vi "EnqueExperiment.vi"(0 "object in":refnum<class "Experiment.lvclass">, 1 "Message":string, 3 "Message Data":variant, 5 "error in (no error)":errorcluster) -> (14 "object out":refnum<class "Experiment.lvclass">, 19 "error out":errorcluster)   [LabVIEW 2023, in "Experiment.lvclass"]
uses:
  Experiment.lvclass
  Experiment.lvclass/Experiment.ctl
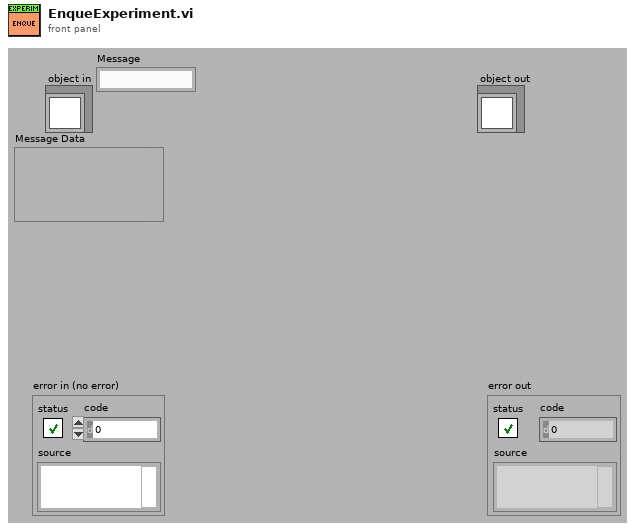
[diagram p1: front panel]
types:
  T1 = cluster{"Message":string, "Message Data":variant}
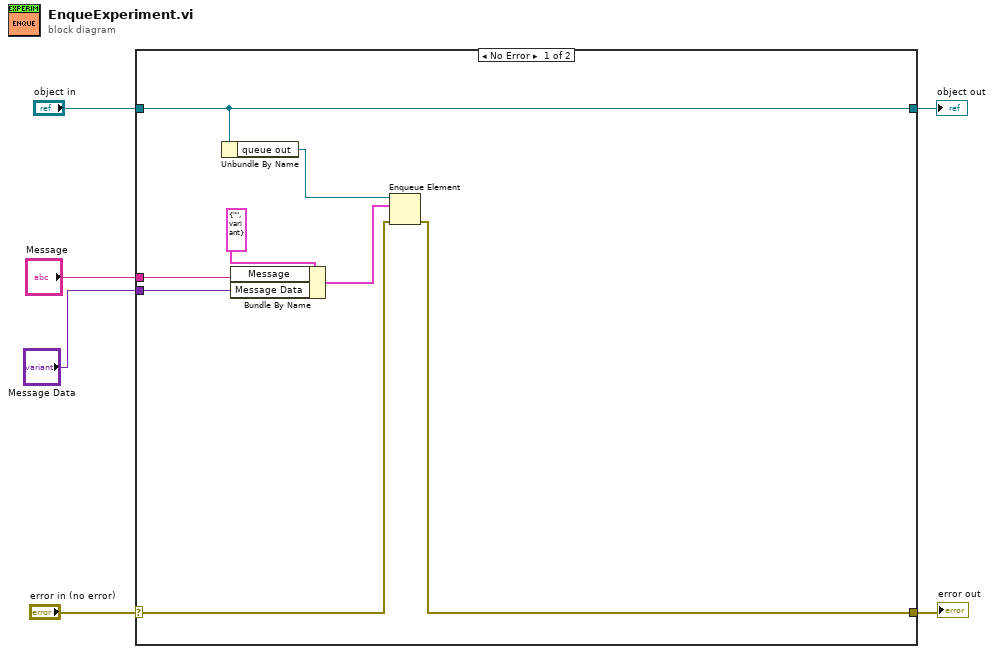
[diagram p0: block diagram]
diagram:
  n1 = case shown="No Error" "error in (no error)" {
    selector: "error in (no error)" -> [w12 w16]
    tunnel: [w11 w16] -> w5
    tunnel: [w14 w15] -> w3
    tunnel: "object in" -> [w14 w15]
    tunnel: "Message" -> [w9 _]
    tunnel: "Message Data" -> [w7 _]
    frame No Error {
      n2 = Unbundle By Name(w14) -> ("queue out"=w13:refnum<queue>)
      n3 = Bundle By Name(cluster=T1 {"Message"="", "Message Data"=variant} ("element"), "Message"=w9, "Message Data"=w7) -> (w8:T1)
      n4 = Enqueue Element(queue=w13, element=w8, error in (no error)=w12) -> (error out=w11:errorcluster)  [unwired: 1 in, 2 out]
    }
    frame Error {
    }
  }
  "error out" <- w5
  "object out" <- w3
